vi "Info.vi"(8 "Error In":errorcluster, 11 "Command":string) -> (0 "Error Out":errorcluster, 3 "Response":string)   [LabVIEW 2018]
uses:
  MOKO_LabViewLibrary/MokoLowLevel/MokoLowLovelControl/MLLC_Mode.ctl
  windows/Info_Equipment.ctl
  windows/Info_Environments.ctl
  windows/Info_Registration.ctl
panel:
  in  "Settings":T4
  in  "Error Code":u32
  in  "Utility Name":string="Info"
  in  "Mode":T5
  # "Temporary data"
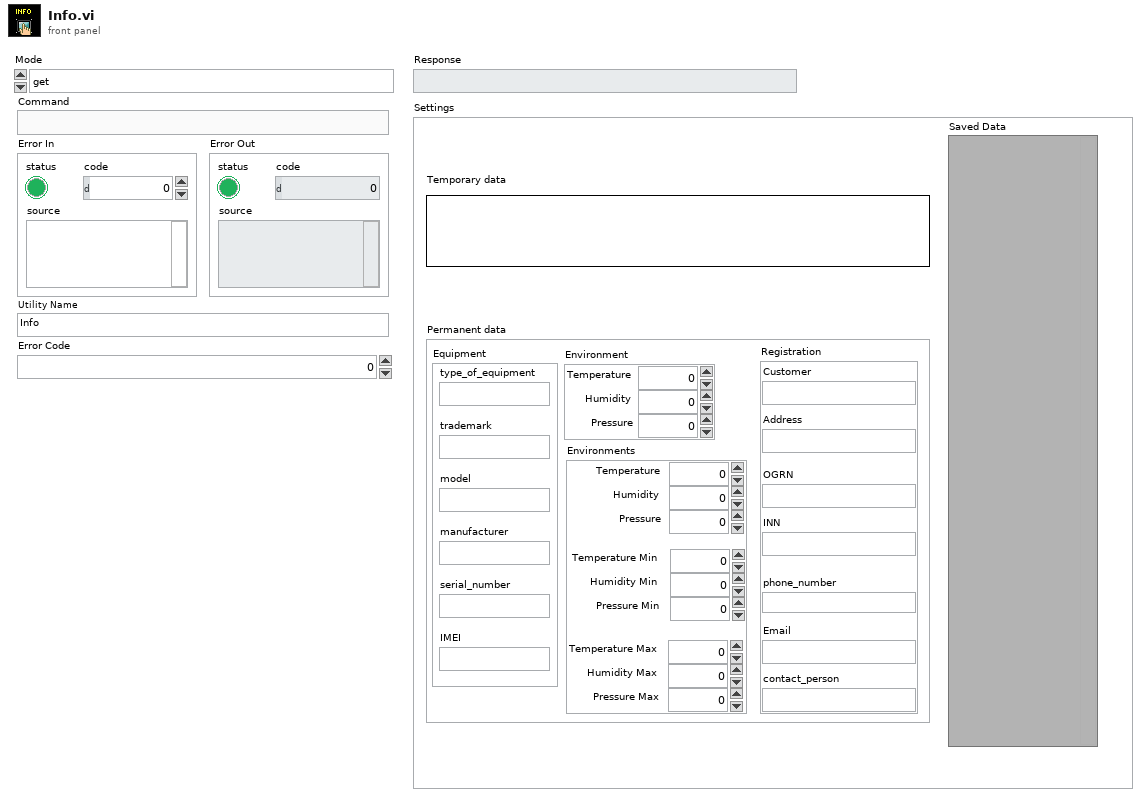
[diagram p1: front panel]
types:
  T1 = typedef "Info_Equipment.ctl" = cluster{"type_of_equipment":string, "trademark":string, "model":string, "manufacturer":string, "serial_number":string, "IMEI":string}
  T2 = typedef "Info_Environments.ctl" = cluster{"Temperature Min":dbl, "Humidity Min":dbl, "Pressure Min":dbl, "Temperature Max":dbl, "Humidity Max":dbl, "Pressure Max":dbl, "Temperature":dbl, "Humidity":dbl, "Pressure":dbl}
  T3 = typedef "Info_Registration.ctl" = cluster{"name_of_the_customer":string, "the_address_of_the_customer":string, "OGRN":string, "INN":string, "phone_number":string, "Email":string, "contact_person":string}
  T4 = cluster{"Saved Data":variant, "Permanent data":cluster{"Equipment":T1, "Environment":cluster{"Temperature":dbl, "Humidity":dbl, "Pressure":dbl}, "Environments":T2, "Registration":T3}}
  T5 = typedef "MLLC_Mode.ctl" = enum16{"get", "set", "close", "Init", "Check"}
  T6 = cluster{"Equipment":T1, "Environment":cluster{"Temperature":dbl, "Humidity":dbl, "Pressure":dbl}, "Environments":T2, "Registration":T3}
  T7 = cluster{"Temperature":dbl, "Humidity":dbl, "Pressure":dbl}
  T8 = typedef "MLLC_Error.ctl" = errorcluster
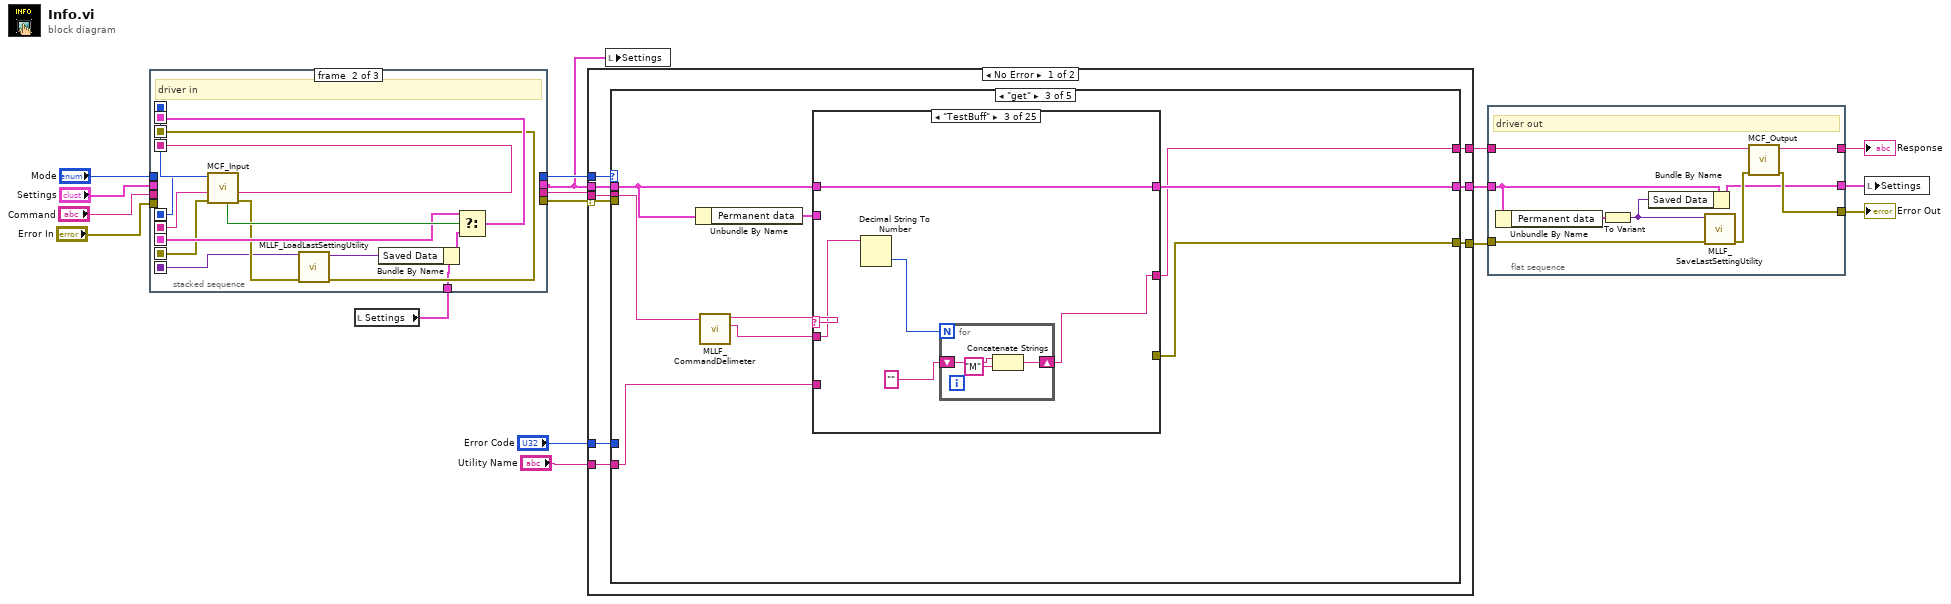
[diagram p0: block diagram]
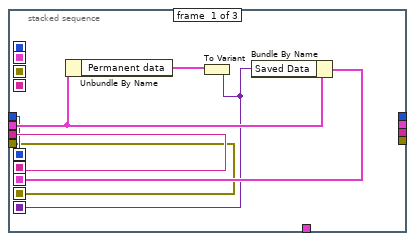
[diagram p2: hidden frame]
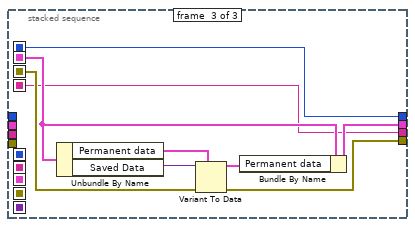
[diagram p3: hidden frame]
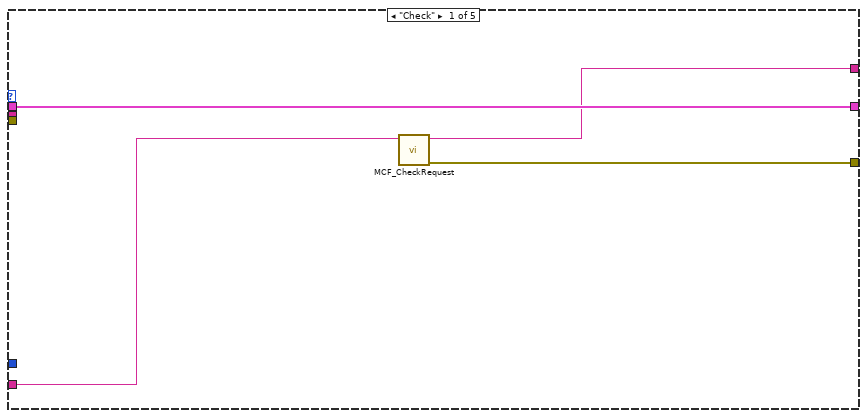
[diagram p4: hidden frame]
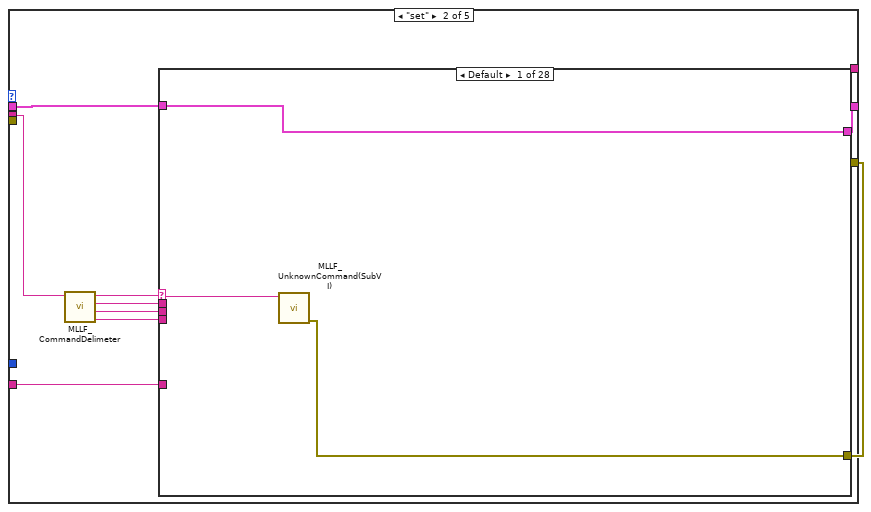
[diagram p5: hidden frame]
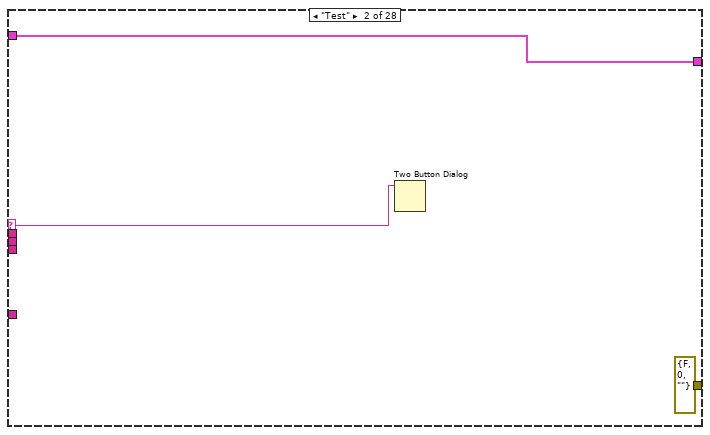
[diagram p6: hidden frame]
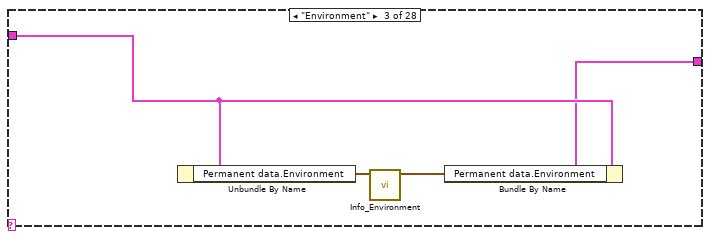
[diagram p7: hidden frame]
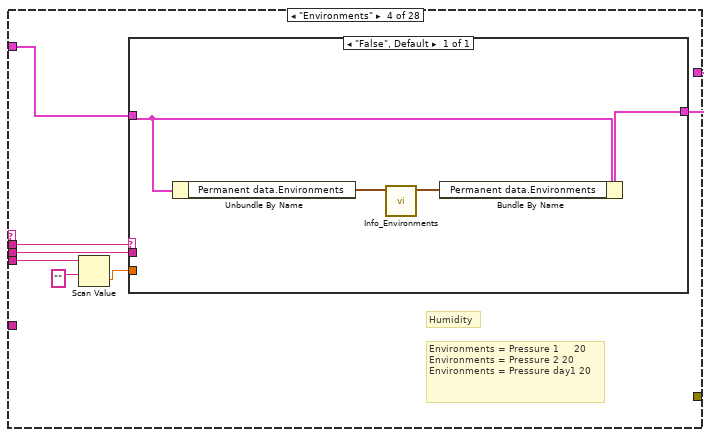
[diagram p8: hidden frame]
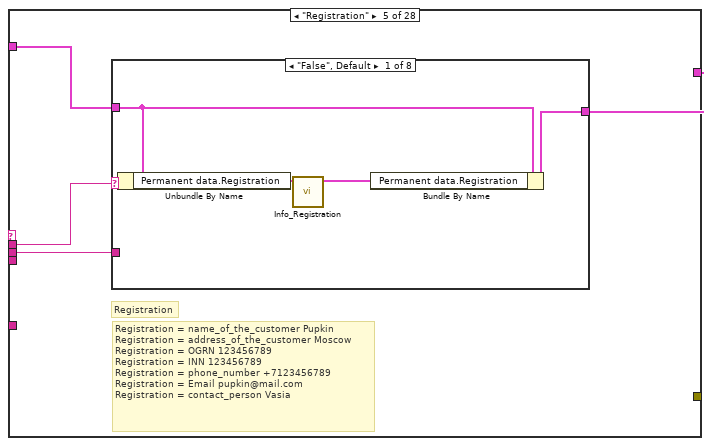
[diagram p9: hidden frame]
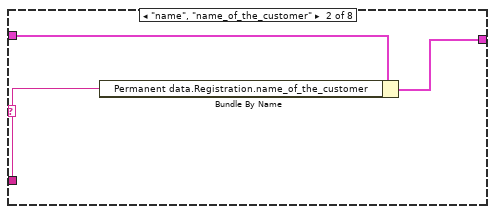
[diagram p10: hidden frame]
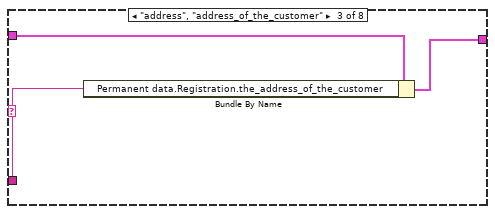
[diagram p11: hidden frame]
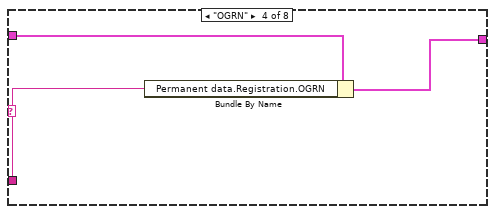
[diagram p12: hidden frame]
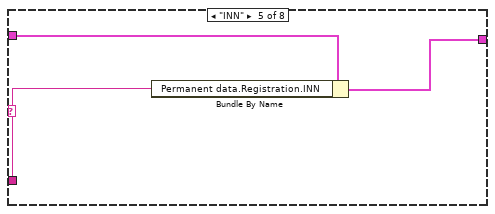
[diagram p13: hidden frame]
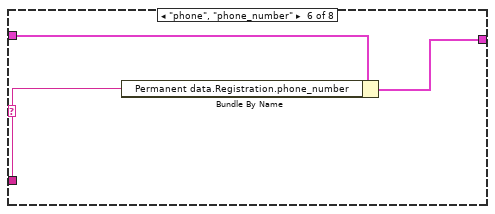
[diagram p14: hidden frame]
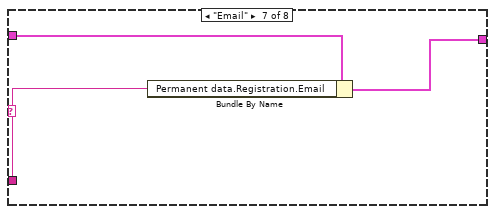
[diagram p15: hidden frame]
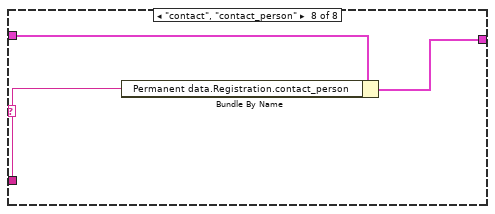
[diagram p16: hidden frame]
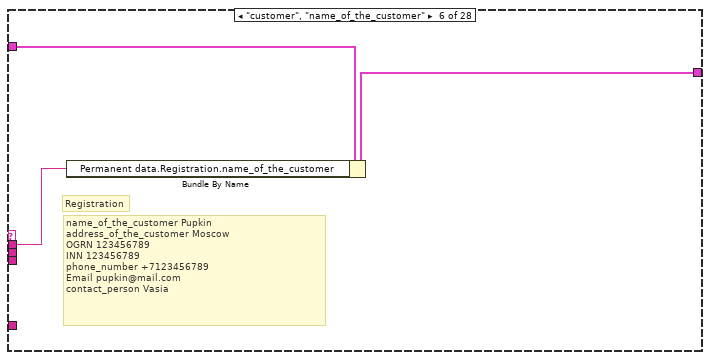
[diagram p17: hidden frame]
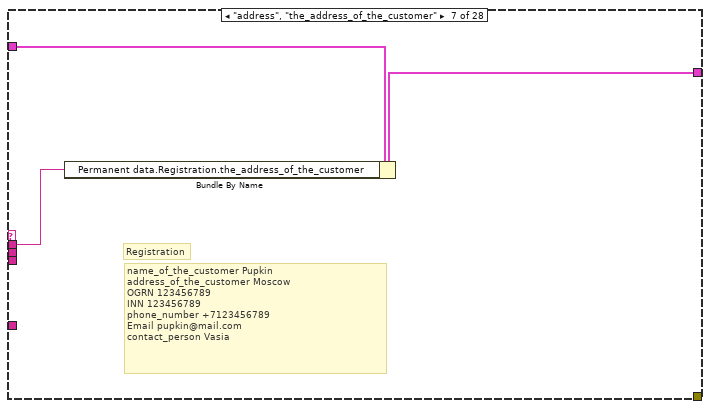
[diagram p18: hidden frame]
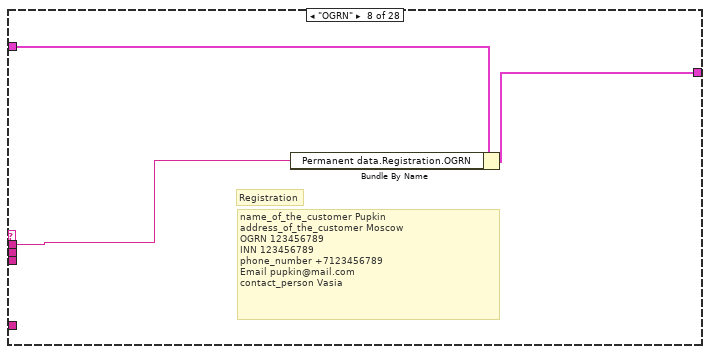
[diagram p19: hidden frame]
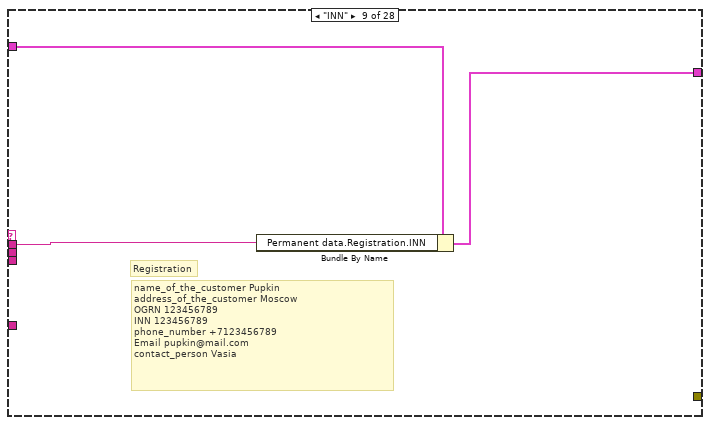
[diagram p20: hidden frame]
diagram:
  n1 = local read "Settings"() -> (w7:T4)
  n2 = stacked-sequence {
    seq-local: [w20 _ _] -> [_ w36 _]
    seq-local: [w19 _ _] -> [_ w37 _]
    seq-local: [w22 _ _] -> [_ w32 _]
    seq-local: [w18 _ _] -> [_ w31 _]
    seq-local: [w21 _ _] -> [_ w26 _]
    seq-local: [_ w27 _] -> [_ _ w43]
    seq-local: [_ w38 _] -> [_ _ w40]
    seq-local: [_ w35 _] -> [_ _ w39]
    seq-local: [_ w34 _] -> [_ _ w44]
    tunnel: "Command" -> [w20 _ _]
    tunnel: "Mode" -> [w19 _ _]
    tunnel: "Error In" -> [w18 _ _]
    tunnel: "Settings" -> [w23 _ _]
    tunnel: w7 -> [_ w25 _]
    tunnel: [_ _ w39] -> w9
    tunnel: [_ _ w42] -> w10
    tunnel: [_ _ w41] -> w8
    tunnel: [_ _ w40] -> w11
    frame #0 {
      n3 = Unbundle By Name(w23) -> ("Permanent data"=w24:T6)
      n4 = To Variant(anything=w24) -> (Variant=w21:variant)
      n5 = Bundle By Name(cluster=w23, "Saved Data"=w21) -> (w22:T4)
    }
    frame #1 {
      # "driver in"
      n6 = call "MCF_Input.vi"("Error In"=w31, "Command in"=w36, "Mode in"=w37) -> ("Error Out"=w30:errorcluster, "Command out"=w35:string, "Mode out"=w38:T5, "Boolean"=w33:bool)  [unwired: 5 in]
      n7 = call "MLLF_LoadLastSettingUtility.vi"("Error In"=w30, "Save data in"=w26) -> ("Error Out"=w27:errorcluster, "Save data out"=w29:variant)  [unwired: 8 in]
      n8 = Bundle By Name(cluster=w25, "Saved Data"=w29) -> (w28:T4)
      n9 = Select(t=w32, s=w33, f=w28) -> (s? t:f=w34:T4)
    }
    frame #2 {
      n10 = Unbundle By Name(w44) -> ("Permanent data"=w45:T6, "Saved Data"=w47:variant)
      n11 = Variant To Data(error in=w43, type=w45, Variant=w47) -> (data=w46:T6, error out=w41:errorcluster)
      n12 = Bundle By Name(cluster=w44, "Permanent data"=w46) -> (w42:T4)
    }
  }
  n13 = case shown="No Error" w8 {
    selector: w8 -> [w52 w329]
    tunnel: [w54 w329] -> w4
    tunnel: w11 -> [w56 _]
    tunnel: [w55 _] -> w6
    tunnel: w9 -> [w53 _]
    tunnel: w10 -> [w49 w328]
    tunnel: "Error Code" -> [w51 _]
    tunnel: "Utility Name" -> [w50 _]
    tunnel: [w48 w328] -> w5
    frame No Error {
      n14 = case shown="\"get\"" w56 {
        tunnel: [w58 _ w210 _ _] -> w55
        tunnel: [w57 w68 w213 _ _] -> w54
        tunnel: w53 -> [_ w69 w216 _ _]
        tunnel: w52 -> [_ _ _ _ _]
        tunnel: w51 -> [_ _ _ _ _]
        tunnel: w50 -> [w59 w61 w209 _ _]
        tunnel: w49 -> [w60 w67 w215 _ w327]
        tunnel: [w60 w66 w214 _ w327] -> w48
        frame "Check" {
          n15 = call "MCF_CheckRequest.vi"("Driver Name"=w59) -> ("Error Out"=w57:errorcluster, "Output String"=w58:string)  [unwired: 9 in]
        }
        frame "set" {
          # "Тут реализованы функции DriverSet"
          n16 = call "MLLF_CommandDelimeter.vi"("command with param"=w69) -> ("param 3"=w62:string, "param 2"=w63:string, "param 1"=w64:string, "command"=w65:string)  [unwired: 6 in, 1 out]
          n17 = case shown="Default" w65 {
            selector: w65 -> [w71 w73 _ _ _ _ _ _ _ _ _ _ _ _ _ _ _ _ _ _ _ _ _ _ _ _ _ _]
            tunnel: [w72 w75 w77 w85 w93 w121 w124 w127 w130 w133 w136 w139 w141 w146 w149 w152 w155 w158 w161 w166 w171 w176 w181 w186 w191 w196 w201 w206] -> w66
            tunnel: w67 -> [w72 w75 w78 w86 w94 w122 w125 w128 w131 w134 w137 w140 w143 w147 w150 w153 w156 w159 w162 w167 w172 w177 w182 w187 w192 w197 w202 w207]
            tunnel: [w70 errorcluster {"status"=FALSE, "code"=0, "source"=""} ("error IO") _ _ _ _ _ _ _ _ _ _ _ _ _ _ _ _ _ _ _ _ _ _ _ _ _ _] -> w68
            tunnel: w64 -> [_ _ _ w82 w92 w120 w123 w126 w129 w132 w135 w138 _ w145 w148 w151 w154 w157 w160 w163 w168 w173 w178 w183 w188 w193 w198 w203]
            tunnel: w63 -> [_ _ _ w81 w91 _ _ _ _ _ _ _ _ _ _ _ _ _ _ _ _ _ _ _ _ _ _ _]
            tunnel: w62 -> [_ _ _ w80 _ _ _ _ _ _ _ _ _ _ _ _ _ _ _ _ _ _ _ _ _ _ _ _]
            tunnel: w61 -> [_ _ _ _ _ _ _ _ _ _ _ _ _ _ _ _ _ _ _ _ _ _ _ _ _ _ _ _]
            frame Default {
              n18 = call "MLLF_UnknownCommand(SubVI).vi"("Unknown command"=w71) -> ("error out"=w70:errorcluster)  [unwired: 10 in]
            }
            frame "Test" {
              n19 = Two Button Dialog(message=w73) -> ()  [unwired: 2 in, 1 out]
            }
            frame "Environment" {
              n20 = Unbundle By Name(w78) -> ("Permanent data.Environment"=w79:T7)
              n21 = call "Info_Environment.vi"("Environment in"=w79) -> ("Environment out"=w76:T7)  [unwired: 9 in, 1 out]
              n22 = Bundle By Name(cluster=w78, "Permanent data.Environment"=w76) -> (w77:T4)
            }
            frame "Environments" {
              # "Humidity"
              # "Environments = Pressure 1     20\nEnvironments = Pressure 2 20\nEnvironments = Pressure day1 20"
              n23 = Scan Value(string=w80, format string="") -> (value=w84:dbl)  [unwired: 1 in, 1 out]
              n24 = case shown="\"False\", Default" w82 {
                tunnel: w86 -> [w88]
                tunnel: [w87] -> w85
                tunnel: w84 -> [_]
                tunnel: w81 -> [_]
                frame "False", Default {
                  n25 = Unbundle By Name(w88) -> ("Permanent data.Environments"=w90:T2)
                  n26 = call "Info_Environments.vi"("Environments in"=w90) -> ("Environments out"=w89:T2)  [unwired: 9 in, 1 out]
                  n27 = Bundle By Name(cluster=w88, "Permanent data.Environments"=w89) -> (w87:T4)
                }
              }
            }
            frame "Registration" {
              # "Registration"
              # "Registration = name_of_the_customer Pupkin\nRegistration = address_of_the_customer Moscow\nRegistration = OGRN 123456789\nRegistration = INN 123456789\nRegistration = phone_number +7123456789\nRegistration = Email pupkin@mail.com\nRegistration = contact_person Vasia"
              n28 = case shown="\"False\", Default" w92 {
                tunnel: w94 -> [w97 w101 w104 w107 w110 w113 w116 w119]
                tunnel: [w96 w100 w103 w106 w109 w112 w115 w118] -> w93
                tunnel: w91 -> [_ w99 w102 w105 w108 w111 w114 w117]
                frame "False", Default {
                  n29 = Unbundle By Name(w97) -> ("Permanent data.Registration"=w98:T3)
                  n30 = call "Info_Registration.vi"("Registration in"=w98) -> ("Registration out"=w95:T3)  [unwired: 9 in, 1 out]
                  n31 = Bundle By Name(cluster=w97, "Permanent data.Registration"=w95) -> (w96:T4)
                }
                frame "name", "name_of_the_customer" {
                  n32 = Bundle By Name(cluster=w101, "Permanent data.Registration.name_of_the_customer"=w99) -> (w100:T4)
                }
                frame "address", "address_of_the_customer" {
                  n33 = Bundle By Name(cluster=w104, "Permanent data.Registration.the_address_of_the_customer"=w102) -> (w103:T4)
                }
                frame "OGRN" {
                  n34 = Bundle By Name(cluster=w107, "Permanent data.Registration.OGRN"=w105) -> (w106:T4)
                }
                frame "INN" {
                  n35 = Bundle By Name(cluster=w110, "Permanent data.Registration.INN"=w108) -> (w109:T4)
                }
                frame "phone", "phone_number" {
                  n36 = Bundle By Name(cluster=w113, "Permanent data.Registration.phone_number"=w111) -> (w112:T4)
                }
                frame "Email" {
                  n37 = Bundle By Name(cluster=w116, "Permanent data.Registration.Email"=w114) -> (w115:T4)
                }
                frame "contact", "contact_person" {
                  n38 = Bundle By Name(cluster=w119, "Permanent data.Registration.contact_person"=w117) -> (w118:T4)
                }
              }
            }
            frame "customer", "name_of_the_customer" {
              # "Registration"
              # "name_of_the_customer Pupkin\naddress_of_the_customer Moscow\nOGRN 123456789\nINN 123456789\nphone_number +7123456789\nEmail pupkin@mail.com\ncontact_person Vasia"
              n39 = Bundle By Name(cluster=w122, "Permanent data.Registration.name_of_the_customer"=w120) -> (w121:T4)
            }
            frame "address", "the_address_of_the_customer" {
              # "Registration"
              # "name_of_the_customer Pupkin\naddress_of_the_customer Moscow\nOGRN 123456789\nINN 123456789\nphone_number +7123456789\nEmail pupkin@mail.com\ncontact_person Vasia"
              n40 = Bundle By Name(cluster=w125, "Permanent data.Registration.the_address_of_the_customer"=w123) -> (w124:T4)
            }
            frame "OGRN" {
              # "Registration"
              # "name_of_the_customer Pupkin\naddress_of_the_customer Moscow\nOGRN 123456789\nINN 123456789\nphone_number +7123456789\nEmail pupkin@mail.com\ncontact_person Vasia"
              n41 = Bundle By Name(cluster=w128, "Permanent data.Registration.OGRN"=w126) -> (w127:T4)
            }
            frame "INN" {
              # "Registration"
              # "name_of_the_customer Pupkin\naddress_of_the_customer Moscow\nOGRN 123456789\nINN 123456789\nphone_number +7123456789\nEmail pupkin@mail.com\ncontact_person Vasia"
              n42 = Bundle By Name(cluster=w131, "Permanent data.Registration.INN"=w129) -> (w130:T4)
            }
            frame "phone", "phone_number" {
              # "Registration"
              # "name_of_the_customer Pupkin\naddress_of_the_customer Moscow\nOGRN 123456789\nINN 123456789\nphone_number +7123456789\nEmail pupkin@mail.com\ncontact_person Vasia"
              n43 = Bundle By Name(cluster=w134, "Permanent data.Registration.phone_number"=w132) -> (w133:T4)
            }
            frame "Email" {
              # "Registration"
              # "name_of_the_customer Pupkin\naddress_of_the_customer Moscow\nOGRN 123456789\nINN 123456789\nphone_number +7123456789\nEmail pupkin@mail.com\ncontact_person Vasia"
              n44 = Bundle By Name(cluster=w137, "Permanent data.Registration.Email"=w135) -> (w136:T4)
            }
            frame "contact", "contact_person" {
              # "Registration"
              # "name_of_the_customer Pupkin\naddress_of_the_customer Moscow\nOGRN 123456789\nINN 123456789\nphone_number +7123456789\nEmail pupkin@mail.com\ncontact_person Vasia"
              n45 = Bundle By Name(cluster=w140, "Permanent data.Registration.contact_person"=w138) -> (w139:T4)
            }
            frame "Equipment" {
              n46 = Unbundle By Name(w143) -> ("Permanent data.Equipment"=w144:T1)
              n47 = call "Info_Equipment.vi"("Equipment in"=w144) -> ("Equipment out"=w142:T1)  [unwired: 9 in, 1 out]
              n48 = Bundle By Name(cluster=w143, "Permanent data.Equipment"=w142) -> (w141:T4)
            }
            frame "type_of_equipment" {
              # "Equipment"
              # "type_of_equipment Reciever\ntrademark Roga&Kopyta\nmodel Model_1\nmanufacturer Roga&Kopyta\nserial_number 123456789\nIMEI 55613216568486483465"
              n49 = Bundle By Name(cluster=w147, "Permanent data.Equipment.type_of_equipment"=w145) -> (w146:T4)
            }
            frame "trademark" {
              # "Equipment"
              # "type_of_equipment Reciever\ntrademark Roga&Kopyta\nmodel Model_1\nmanufacturer Roga&Kopyta\nserial_number 123456789\nIMEI 55613216568486483465"
              n50 = Bundle By Name(cluster=w150, "Permanent data.Equipment.trademark"=w148) -> (w149:T4)
            }
            frame "model" {
              # "Equipment"
              # "type_of_equipment Reciever\ntrademark Roga&Kopyta\nmodel Model_1\nmanufacturer Roga&Kopyta\nserial_number 123456789\nIMEI 55613216568486483465"
              n51 = Bundle By Name(cluster=w153, "Permanent data.Equipment.model"=w151) -> (w152:T4)
            }
            frame "manufacturer" {
              # "Equipment"
              # "type_of_equipment Reciever\ntrademark Roga&Kopyta\nmodel Model_1\nmanufacturer Roga&Kopyta\nserial_number 123456789\nIMEI 55613216568486483465"
              n52 = Bundle By Name(cluster=w156, "Permanent data.Equipment.manufacturer"=w154) -> (w155:T4)
            }
            frame "serial_number" {
              # "Equipment"
              # "type_of_equipment Reciever\ntrademark Roga&Kopyta\nmodel Model_1\nmanufacturer Roga&Kopyta\nserial_number 123456789\nIMEI 55613216568486483465"
              n53 = Bundle By Name(cluster=w159, "Permanent data.Equipment.serial_number"=w157) -> (w158:T4)
            }
            frame "IMEI" {
              # "Equipment"
              # "type_of_equipment Reciever\ntrademark Roga&Kopyta\nmodel Model_1\nmanufacturer Roga&Kopyta\nserial_number 123456789\nIMEI 55613216568486483465"
              n54 = Bundle By Name(cluster=w162, "Permanent data.Equipment.IMEI"=w160) -> (w161:T4)
            }
            frame "Temperature" {
              # "Enviroments"
              # "Temperature 25\nHumidity 50\nPressure 100\nTemperature_min 25\nHumidity_min 50\nPressure_min 100\nTemperature_max 25\nHumidity_max 50\nPressure_max 100"
              n55 = Scan Value(string=w163, format string="") -> (value=w165:dbl)  [unwired: 1 in, 1 out]
              n56 = Bundle By Name(cluster=w167, "Permanent data.Environment.Temperature"=w165) -> (w166:T4)
            }
            frame "Humidity" {
              # "Enviroments"
              # "Temperature 25\nHumidity 50\nPressure 100\nTemperature_min 25\nHumidity_min 50\nPressure_min 100\nTemperature_max 25\nHumidity_max 50\nPressure_max 100"
              n57 = Scan Value(string=w168, format string="") -> (value=w170:dbl)  [unwired: 1 in, 1 out]
              n58 = Bundle By Name(cluster=w172, "Permanent data.Environment.Humidity"=w170) -> (w171:T4)
            }
            frame "Pressure" {
              # "Enviroments"
              # "Temperature 25\nHumidity 50\nPressure 100\nTemperature_min 25\nHumidity_min 50\nPressure_min 100\nTemperature_max 25\nHumidity_max 50\nPressure_max 100"
              n59 = Scan Value(string=w173, format string="") -> (value=w175:dbl)  [unwired: 1 in, 1 out]
              n60 = Bundle By Name(cluster=w177, "Permanent data.Environment.Pressure"=w175) -> (w176:T4)
            }
            frame "Temperature_min", "TemperatureMin" {
              # "Enviroments"
              # "Temperature 25\nHumidity 50\nPressure 100\nTemperature_min 25\nHumidity_min 50\nPressure_min 100\nTemperature_max 25\nHumidity_max 50\nPressure_max 100"
              n61 = Scan Value(string=w178, format string="") -> (value=w180:dbl)  [unwired: 1 in, 1 out]
              n62 = Bundle By Name(cluster=w182, "Permanent data.Environments.Temperature Min"=w180) -> (w181:T4)
            }
            frame "Humidity_min", "HumidityMin" {
              # "Enviroments"
              # "Temperature 25\nHumidity 50\nPressure 100\nTemperature_min 25\nHumidity_min 50\nPressure_min 100\nTemperature_max 25\nHumidity_max 50\nPressure_max 100"
              n63 = Scan Value(string=w183, format string="") -> (value=w185:dbl)  [unwired: 1 in, 1 out]
              n64 = Bundle By Name(cluster=w187, "Permanent data.Environments.Humidity Min"=w185) -> (w186:T4)
            }
            frame "Pressure_min", "PressureMin" {
              # "Enviroments"
              # "Temperature 25\nHumidity 50\nPressure 100\nTemperature_min 25\nHumidity_min 50\nPressure_min 100\nTemperature_max 25\nHumidity_max 50\nPressure_max 100"
              n65 = Scan Value(string=w188, format string="") -> (value=w190:dbl)  [unwired: 1 in, 1 out]
              n66 = Bundle By Name(cluster=w192, "Permanent data.Environments.Pressure Min"=w190) -> (w191:T4)
            }
            frame "Temperature_max", "TemperatureMax" {
              # "Enviroments"
              # "Temperature 25\nHumidity 50\nPressure 100\nTemperature_min 25\nHumidity_min 50\nPressure_min 100\nTemperature_max 25\nHumidity_max 50\nPressure_max 100"
              n67 = Scan Value(string=w193, format string="") -> (value=w195:dbl)  [unwired: 1 in, 1 out]
              n68 = Bundle By Name(cluster=w197, "Permanent data.Environments.Temperature Max"=w195) -> (w196:T4)
            }
            frame "Humidity_max", "HumidityMax" {
              # "Enviroments"
              # "Temperature 25\nHumidity 50\nPressure 100\nTemperature_min 25\nHumidity_min 50\nPressure_min 100\nTemperature_max 25\nHumidity_max 50\nPressure_max 100"
              n69 = Scan Value(string=w198, format string="") -> (value=w200:dbl)  [unwired: 1 in, 1 out]
              n70 = Bundle By Name(cluster=w202, "Permanent data.Environments.Humidity Max"=w200) -> (w201:T4)
            }
            frame "Pressure_max", "PressureMax" {
              # "Enviroments"
              # "Temperature 25\nHumidity 50\nPressure 100\nTemperature_min 25\nHumidity_min 50\nPressure_min 100\nTemperature_max 25\nHumidity_max 50\nPressure_max 100"
              n71 = Scan Value(string=w203, format string="") -> (value=w205:dbl)  [unwired: 1 in, 1 out]
              n72 = Bundle By Name(cluster=w207, "Permanent data.Environments.Pressure Max"=w205) -> (w206:T4)
            }
          }
        }
        frame "get" {
          # "Тут реализованы функции DriverGet"
          n73 = Unbundle By Name(w215) -> ("Permanent data"=w211:T6)
          n74 = call "MLLF_CommandDelimeter.vi"("command with param"=w216) -> ("param 1"=w208:string, "command"=w212:string)  [unwired: 6 in, 3 out]
          n75 = case shown="\"TestBuff\"" w212 {
            selector: w212 -> [w218 _ _ _ _ _ _ _ _ _ _ _ _ _ _ _ _ _ _ _ _ _ _ _ _]
            tunnel: w215 -> [w219 w225 w230 w238 w241 w247 w253 w259 w265 w271 w277 w283 w290 w293 w296 w299 w302 w305 w308 w311 w314 w317 w320 w323 w326]
            tunnel: [w219 w225 w230 w238 w241 w247 w253 w259 w265 w271 w277 w283 w290 w293 w296 w299 w302 w305 w308 w311 w314 w317 w320 w323 w326] -> w214
            tunnel: [_ w220 w226 w234 w240 w246 w252 w258 w264 w270 w276 w282 w288 w292 w295 w298 w301 w304 w307 w310 w313 w316 w319 w322 w325] -> w210
            tunnel: [w217 _ _ _ _ _ _ _ _ _ _ _ _ _ _ _ _ _ _ _ _ _ _ _ _] -> w213
            tunnel: w211 -> [_ _ _ _ _ _ _ _ _ _ _ _ _ _ _ _ _ _ _ _ _ _ _ _ _]
            tunnel: w209 -> [_ _ _ _ _ _ _ _ _ _ _ _ _ _ _ _ _ _ _ _ _ _ _ _ _]
            tunnel: w208 -> [_ _ w229 _ _ _ _ _ _ _ _ _ _ _ _ _ _ _ _ _ _ _ _ _ _]
            frame Default {
              n76 = call "MLLF_UnknownCommand(SubVI).vi"("Unknown command"=w218) -> ("error out"=w217:errorcluster)  [unwired: 10 in]
            }
            frame "Test" {
              n77 = Two Button Dialog(message="Test") -> (T button?=w224:bool)  [unwired: 2 in]
              n78 = Select(t="True" ("string"), s=w224, f="False" ("string")) -> (s? t:f=w220:string)
            }
            frame "TestBuff" {
              n79 = Decimal String To Number(string=w229) -> (number=w228:i32)  [unwired: 2 in, 1 out]
              n80 = for {
                N: w228 -> [_]
                shift-right: [w232] -> w226
                shift-left: "" -> [w233]
                n81 = Concatenate Strings(w233, "M" ("string")) -> (w232:string)
              }
            }
            frame "Temperature" {
              n82 = Unbundle By Name(w238) -> ("Permanent data.Environment.Temperature"=w239:dbl)
              n83 = Format Value(value (0)=w239) -> (output string=w237:string)  [unwired: 2 in]
              n84 = Search and Replace String(input string=w237, search string=",", replace string="." ("replace string (\"\")")) -> (result string=w234:string)  [unwired: 5 in, 3 out]
            }
            frame "Humidity" {
              n85 = Unbundle By Name(w241) -> ("Permanent data.Environment.Humidity"=w245:dbl)
              n86 = Format Value(value (0)=w245) -> (output string=w244:string)  [unwired: 2 in]
              n87 = Search and Replace String(input string=w244, search string=",", replace string="." ("replace string (\"\")")) -> (result string=w240:string)  [unwired: 5 in, 3 out]
            }
            frame "Pressure" {
              n88 = Unbundle By Name(w247) -> ("Permanent data.Environment.Pressure"=w251:dbl)
              n89 = Format Value(value (0)=w251) -> (output string=w250:string)  [unwired: 2 in]
              n90 = Search and Replace String(input string=w250, search string=",", replace string="." ("replace string (\"\")")) -> (result string=w246:string)  [unwired: 5 in, 3 out]
            }
            frame "Temperature_min", "TemperatureMin" {
              n91 = Unbundle By Name(w253) -> ("Permanent data.Environments.Temperature Min"=w257:dbl)
              n92 = Format Value(value (0)=w257) -> (output string=w256:string)  [unwired: 2 in]
              n93 = Search and Replace String(input string=w256, search string=",", replace string="." ("replace string (\"\")")) -> (result string=w252:string)  [unwired: 5 in, 3 out]
            }
            frame "Humidity_min", "HumidityMin" {
              n94 = Unbundle By Name(w259) -> ("Permanent data.Environments.Humidity Min"=w263:dbl)
              n95 = Format Value(value (0)=w263) -> (output string=w262:string)  [unwired: 2 in]
              n96 = Search and Replace String(input string=w262, search string=",", replace string="." ("replace string (\"\")")) -> (result string=w258:string)  [unwired: 5 in, 3 out]
            }
            frame "Pressure_min", "PressureMin" {
              n97 = Unbundle By Name(w265) -> ("Permanent data.Environments.Pressure Min"=w269:dbl)
              n98 = Format Value(value (0)=w269) -> (output string=w268:string)  [unwired: 2 in]
              n99 = Search and Replace String(input string=w268, search string=",", replace string="." ("replace string (\"\")")) -> (result string=w264:string)  [unwired: 5 in, 3 out]
            }
            frame "Temperature_max", "TemperatureMax" {
              n100 = Unbundle By Name(w271) -> ("Permanent data.Environments.Temperature Max"=w275:dbl)
              n101 = Format Value(value (0)=w275) -> (output string=w274:string)  [unwired: 2 in]
              n102 = Search and Replace String(input string=w274, search string=",", replace string="." ("replace string (\"\")")) -> (result string=w270:string)  [unwired: 5 in, 3 out]
            }
            frame "Humidity_max", "HumidityMax" {
              n103 = Unbundle By Name(w277) -> ("Permanent data.Environments.Humidity Max"=w281:dbl)
              n104 = Format Value(value (0)=w281) -> (output string=w280:string)  [unwired: 2 in]
              n105 = Search and Replace String(input string=w280, search string=",", replace string="." ("replace string (\"\")")) -> (result string=w276:string)  [unwired: 5 in, 3 out]
            }
            frame "Pressure_max", "PressureMax" {
              n106 = Unbundle By Name(w283) -> ("Permanent data.Environments.Pressure Max"=w287:dbl)
              n107 = Format Value(value (0)=w287) -> (output string=w286:string)  [unwired: 2 in]
              n108 = Search and Replace String(input string=w286, search string=",", replace string="." ("replace string (\"\")")) -> (result string=w282:string)  [unwired: 5 in, 3 out]
            }
            frame "customer", "name_of_the_customer" {
              n109 = Unbundle By Name(w290) -> ("Permanent data.Registration.name_of_the_customer"=w289:string)
              n110 = call "MLLF_ReplaceTwoQuotesWithOne.vi"("String in 2"=w289) -> ("Result string"=w288:string)  [unwired: 7 in, 3 out]
            }
            frame "address", "the_address_of_the_customer" {
              n111 = Unbundle By Name(w293) -> ("Permanent data.Registration.the_address_of_the_customer"=w291:string)
              n112 = call "MLLF_ReplaceTwoQuotesWithOne.vi"("String in"=w291) -> ("Result string"=w292:string)  [unwired: 7 in, 3 out]
            }
            frame "OGRN" {
              n113 = Unbundle By Name(w296) -> ("Permanent data.Registration.OGRN"=w294:string)
              n114 = call "MLLF_ReplaceTwoQuotesWithOne.vi"("String in"=w294) -> ("Result string"=w295:string)  [unwired: 7 in, 3 out]
            }
            frame "INN" {
              n115 = Unbundle By Name(w299) -> ("Permanent data.Registration.INN"=w297:string)
              n116 = call "MLLF_ReplaceTwoQuotesWithOne.vi"("String in"=w297) -> ("Result string"=w298:string)  [unwired: 7 in, 3 out]
            }
            frame "phone", "phone_number" {
              n117 = Unbundle By Name(w302) -> ("Permanent data.Registration.phone_number"=w300:string)
              n118 = call "MLLF_ReplaceTwoQuotesWithOne.vi"("String in"=w300) -> ("Result string"=w301:string)  [unwired: 7 in, 3 out]
            }
            frame "Email" {
              n119 = Unbundle By Name(w305) -> ("Permanent data.Registration.Email"=w303:string)
              n120 = call "MLLF_ReplaceTwoQuotesWithOne.vi"("String in"=w303) -> ("Result string"=w304:string)  [unwired: 7 in, 3 out]
            }
            frame "contact", "contact_person" {
              n121 = Unbundle By Name(w308) -> ("Permanent data.Registration.contact_person"=w306:string)
              n122 = call "MLLF_ReplaceTwoQuotesWithOne.vi"("String in"=w306) -> ("Result string"=w307:string)  [unwired: 7 in, 3 out]
            }
            frame "type_of_equipment" {
              n123 = Unbundle By Name(w311) -> ("Permanent data.Equipment.type_of_equipment"=w309:string)
              n124 = call "MLLF_ReplaceTwoQuotesWithOne.vi"("String in"=w309) -> ("Result string"=w310:string)  [unwired: 7 in, 3 out]
            }
            frame "trademark" {
              n125 = Unbundle By Name(w314) -> ("Permanent data.Equipment.trademark"=w312:string)
              n126 = call "MLLF_ReplaceTwoQuotesWithOne.vi"("String in"=w312) -> ("Result string"=w313:string)  [unwired: 7 in, 3 out]
            }
            frame "model" {
              n127 = Unbundle By Name(w317) -> ("Permanent data.Equipment.model"=w315:string)
              n128 = call "MLLF_ReplaceTwoQuotesWithOne.vi"("String in"=w315) -> ("Result string"=w316:string)  [unwired: 7 in, 3 out]
            }
            frame "manufacturer" {
              n129 = Unbundle By Name(w320) -> ("Permanent data.Equipment.manufacturer"=w318:string)
              n130 = call "MLLF_ReplaceTwoQuotesWithOne.vi"("String in"=w318) -> ("Result string"=w319:string)  [unwired: 7 in, 3 out]
            }
            frame "serial_number" {
              n131 = Unbundle By Name(w323) -> ("Permanent data.Equipment.serial_number"=w321:string)
              n132 = call "MLLF_ReplaceTwoQuotesWithOne.vi"("String in"=w321) -> ("Result string"=w322:string)  [unwired: 7 in, 3 out]
            }
            frame "IMEI" {
              n133 = Unbundle By Name(w326) -> ("Permanent data.Equipment.IMEI"=w324:string)
              n134 = call "MLLF_ReplaceTwoQuotesWithOne.vi"("String in"=w324) -> ("Result string"=w325:string)  [unwired: 7 in, 3 out]
            }
          }
        }
        frame "close" {
        }
        frame "Init" {
        }
      }
    }
    frame Error {
    }
  }
  n135 = local write "Settings"(w10) -> ()
  n136 = flat-sequence {
    tunnel: [w338] -> w3
    tunnel: [w337] -> w1
    tunnel: w6 -> [w336]
    tunnel: w4 -> [w335]
    tunnel: w5 -> [w331]
    tunnel: [w333] -> w2
    frame #0 {
      # "driver out"
      n137 = Unbundle By Name(w331) -> ("Permanent data"=w330:T6)
      n138 = To Variant(anything=w330) -> (Variant=w332:variant)
      n139 = Bundle By Name(cluster=w331, "Saved Data"=w332) -> (w333:T4)
      n140 = call "MLLF_SaveLastSettingUtility.vi"("error in"=w335, "Saved Data"=w332) -> ("error out"=w334:T8)  [unwired: 8 in, 1 out]
      n141 = call "MCF_Output.vi"("Error In"=w334, "Input"=w336) -> ("Error Out"=w337:errorcluster, "Output"=w338:string)  [unwired: 8 in]
    }
  }
  n142 = local write "Settings"(w2) -> ()
  "Response" <- w3
  "Error Out" <- w1
